vi "AlazarBoardsInSystemByHandle.vi"(0 "Handle":u64, 1 "error in (no error)":errorcluster) -> (2 "Handle":u64, 3 "Board Count":u32, 5 "error out":errorcluster)   [LabVIEW 2009]
doc: "Return the number of digitizer boards in a board system specified by the handle of its master board."
uses:
  ATSApi.dll
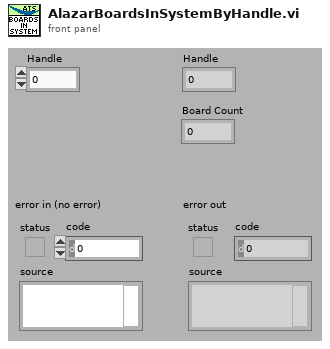
[diagram p1: front panel]
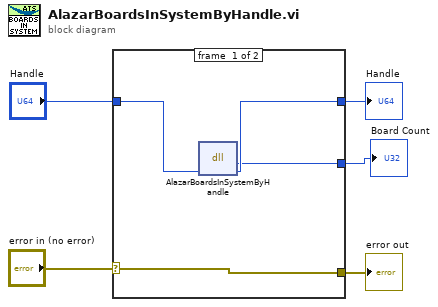
[diagram p0: block diagram]
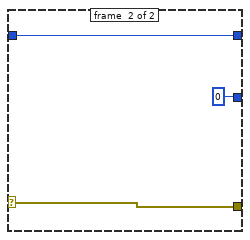
[diagram p2: hidden frame]
diagram:
  n1 = case shown="No Error" "error in (no error)" {
    selector: "error in (no error)" -> [w7 w12]
    tunnel: [w7 w12] -> w4
    tunnel: "Handle" -> [w9 w11]
    tunnel: [w8 w11] -> w2
    tunnel: [w6 u32 0] -> w1
    frame #0 {
      n2 = dll-call lib="ATSApi.dll" fn="AlazarBoardsInSystemByHandle"("handle"=w9) -> ("return type"=w6:u32, "handle"=w8:u64)  [unwired: 3 in, 2 out]
    }
    frame #1 {
    }
  }
  "Handle" <- w2
  "error out" <- w4
  "Board Count" <- w1
